vi "PlLoN_grabber_recovery.vi"(7 "Number of Images":u32=1 min=1 step=1, 8 "error in (no error)":errorcluster, 10 "refnum":refnum<file>, 11 "Camera Handle":u32) -> (0 "error out":errorcluster, 1 "DATA":u16[][](array[numeric]), 2 "Number of Images":u32=1 min=1 step=1, 3 "Camera Handle":u32, 4 "x/y":dbl, 5 "refnum out":refnum<file>, 6 "x > y?":bool, 9 "Frame Rate":dbl=1001.0010010010011)   [LabVIEW 2015]
panel:
  out "Waveform Graph":dbl[][](graph)
  out "PyLoN Ready":bool
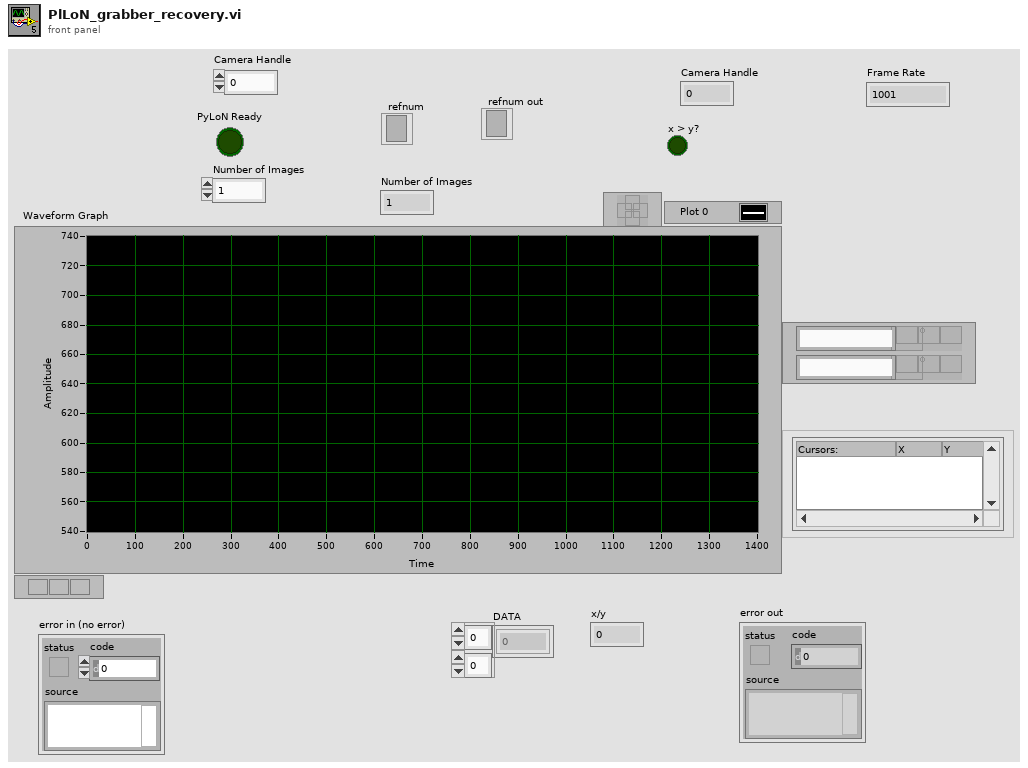
[diagram p1: front panel]
types:
  T1 = cluster{"acquire focus mode":u32, "Exposure Time (s)":dbl, "Number of Images":u32, "Software accumulation":u32}
  T2 = cluster{"Camera Handle":u32, "Pulser Handle":u32, "File Handle":u32, "Display Handle":u32, "Image Handle":u32}
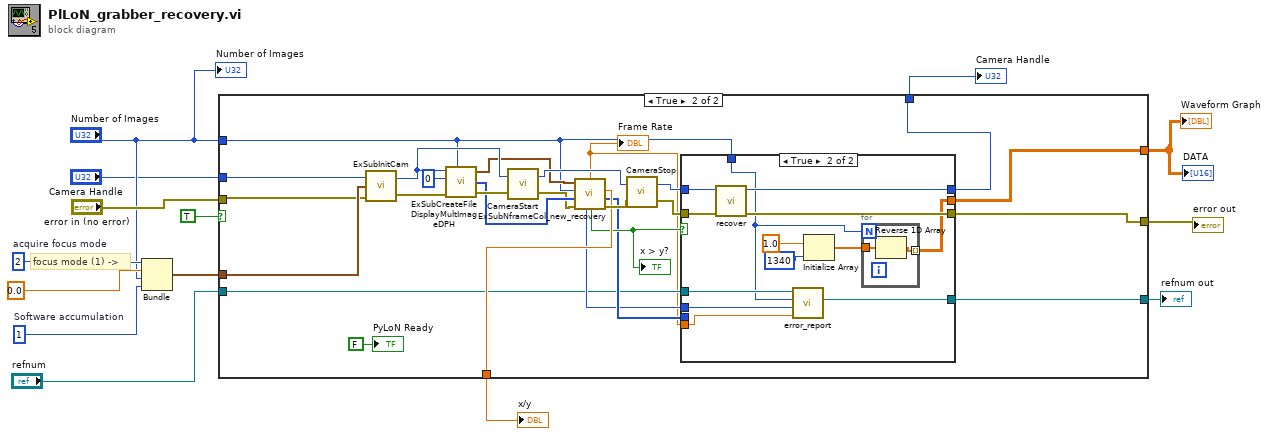
[diagram p0: block diagram]
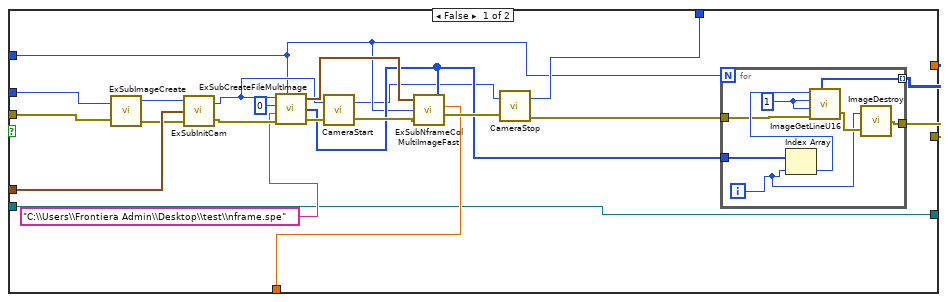
[diagram p2: hidden frame]
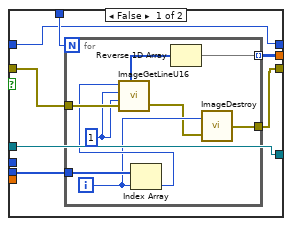
[diagram p3: hidden frame]
diagram:
  w8 = u32 2  # acquire focus mode
  w9 = u32 1  # Software accumulation
  # "focus mode (1) ->"
  n1 = Bundle("acquire focus mode"=w8, "Exposure Time (s)"=0.0, "Number of Images"="Number of Images", "Software accumulation"=w9) -> (w7:T1)  [unwired: 1 in]
  n2 = case shown="True" TRUE {
    tunnel: [w21 w48] -> w3
    tunnel: [w19 w52] -> w14
    tunnel: [w20 w51] -> w13
    tunnel: "Number of Images" -> [w17 w50]
    tunnel: [w18 w59] -> w12
    tunnel: "error in (no error)" -> [w36 w57]
    tunnel: w7 -> [w34 w64]
    tunnel: "Camera Handle" -> [w32 w58]
    tunnel: "refnum" -> [w15 w46]
    tunnel: [w15 w47] -> w1
    frame False {
      n3 = call "ExSubImageCreate.vi"("Camera Handle"=w32, "error in (no error)"=w36) -> ("Camera Handle"=w35:u32, "error out"=w33:errorcluster)  [unwired: 1 out]
      n4 = call "ExSubInitCam.vi"("error in (no error)"=w33, "Camera Information"=w34, "Camera Handle"=w35) -> ("error out"=w31:errorcluster, "Camera Handle"=w25:u32)
      n5 = call "ExSubCreateFileMultImage.vi"("Camera Handle"=w25, "Pulser Handle"=u32 0, "File and Display Name"="C:\\Users\\Frontiera Admin\\Desktop\\test\\nframe.spe", "error in (no error)"=w31, "Number of Images"=w17) -> ("Handles Out"=w26:T2, "Array"=w23:u32[], "error out"=w28:errorcluster)
      n6 = call <userlib>:"CameraStart.vi"("error in"=w28, "Camera Handle"=w25) -> ("error out"=w27:errorcluster, "Camera Handle"=w16:u32)
      n7 = call "ExSubNframeColMultiImageFast.vi"("Handle Cluster"=w26, "Number of Images"=w17, "error in (no error)"=w27, "image handles"=w23) -> ("x/y"=w18:dbl, "error out"=w24:errorcluster)  [unwired: 1 out]
      n8 = call <userlib>:"CameraStop.vi"("error in"=w24, "Camera Handle"=w16) -> ("error out"=w22:errorcluster, "Camera Handle"=w19:u32)
      n9 = for {
        N: w17 -> [_]
        tunnel: w23 -> [w44]
        tunnel: w22 -> [w41]
        tunnel: [w40] -> w21 mode=indexing
        tunnel: [w38] -> w20
        i -> [w37]
        w42 = u32 1 ("Y Position")
        n10 = Index Array(array=w44, index=w37) -> (element=w43:u32)
        n11 = call <userlib>:"ImageGetLineU16.vi"("Data Handle"=w43, "Y Position"=w42, "Z Position"=w42, "error in"=w41) -> ("Array u16"=w40:u16[], "error out"=w39:errorcluster)  [unwired: 1 out]
        n12 = call <userlib>:"ImageDestroy.vi"("error in"=w39, "Data handle"=w37) -> ("error out"=w38:errorcluster)
      }
    }
    frame True {
      n13 = call "ExSubInitCam.vi"("error in (no error)"=w57, "Camera Information"=w64, "Camera Handle"=w58) -> ("error out"=w68:errorcluster, "Camera Handle"=w66:u32)
      n14 = call "ExSubCreateFileDisplayMultImageDPH.vi"("Camera Handle"=w66, "Pulser Handle"=u32 0, "error in (no error)"=w68, "Number of Images"=w50) -> ("Handles Out"=w63:T2, "Array"=w62:u32[], "error out"=w67:errorcluster)  [unwired: 1 in]
      n15 = call <userlib>:"CameraStart.vi"("error in"=w67, "Camera Handle"=w66) -> ("error out"=w61:errorcluster, "Camera Handle"=w69:u32)
      n16 = call "ExSubNframeCol_new_recovery.vi"("error in (no error)"=w61, "image handles"=w62, "Number of Images"=w50, "Handle Cluster 2"=w63) -> ("error out"=w60:errorcluster, "data handles"=w53:u32[], "x/y"=w59:dbl, "x > y?"=w55:bool, "Frame Rate"=w45:dbl, "image #"=w49:i32)  [unwired: 1 in, 1 out]
      "x > y?" <- w55
      "Frame Rate" <- w45
      n17 = call <userlib>:"CameraStop.vi"("error in"=w60, "Camera Handle"=w69) -> ("error out"=w56:errorcluster, "Camera Handle"=w54:u32)
      n18 = case shown="True" w55 {
        tunnel: w56 -> [w76 w97]
        tunnel: [w75 w96] -> w51
        tunnel: w54 -> [w72 w99]
        tunnel: [w72 w98] -> w52
        tunnel: w53 -> [w77 _]
        tunnel: w50 -> [w74 w91]
        tunnel: w49 -> [_ w88]
        tunnel: w46 -> [w71 w93]
        tunnel: [w73 w89] -> w48
        tunnel: [w71 w92] -> w47
        tunnel: w45 -> [_ w87]
        frame False {
          n19 = for {
            N: w74 -> [_]
            tunnel: w77 -> [w83]
            tunnel: w76 -> [w86]
            tunnel: [w78] -> w73 mode=indexing
            tunnel: [w80] -> w75
            i -> [w82]
            w85 = u32 1
            n20 = Index Array(array=w83, index=w82) -> (element=w84:u32)
            n21 = call <userlib>:"ImageGetLineU16.vi"("Data Handle"=w84, "Y Position"=w85, "Z Position"=w85, "error in"=w86) -> ("Array u16"=w79:u16[], "error out"=w81:errorcluster)  [unwired: 1 out]
            n22 = Reverse 1D Array(array=w79) -> (reversed array=w78:u16[])
            n23 = call <userlib>:"ImageDestroy.vi"("error in"=w81, "Data handle"=w82) -> ("error out"=w80:errorcluster)
          }
        }
        frame True {
          n24 = call "recover.vi"("error in (no error)"=w97, "Camera Handle"=w99) -> ("error out"=w96:errorcluster, "Camera Handle"=w98:u32)  [unwired: 7 in, 1 out]
          n25 = call "error_report.vi"("_Frame Rate"=w87, "frame #"=w88, "# of frame"=w91, "refnum"=w93) -> ("refnum out"=w92:refnum<file>)  [unwired: 6 in, 1 out]
          n26 = Initialize Array(1.0 ("element"), 1340 ("dimension size")) -> (w90:dbl[])
          n27 = for {
            N: w91 -> [_]
            tunnel: w90 -> [w100]
            tunnel: [w101] -> w89 mode=indexing
            n28 = Reverse 1D Array(array=w100) -> (reversed array=w101:dbl[])
          }
        }
      }
      "PyLoN Ready" <- FALSE ("PyLoN Ready")
    }
  }
  "error out" <- w13
  "DATA" <- w3
  "Camera Handle" <- w14
  "x/y" <- w12
  "Waveform Graph" <- w3
  "refnum out" <- w1
  "Number of Images" <- "Number of Images"
